vi "DLL Retcode to VI Errcode.vi"(8 "error in (no error)":errorcluster, 10 "Function Name":T1, 11 "DLL Retcode":i32 format="%x") -> (0 "error out":errorcluster, 2 "ErrorMessage":string, 3 "VI Errcode":i32 format="%x")   [LabVIEW 2020, in "Keyence CL-3000.lvlib"]
uses:
  Keyence CL-3000.lvlib
  enums/Function Name.ctl
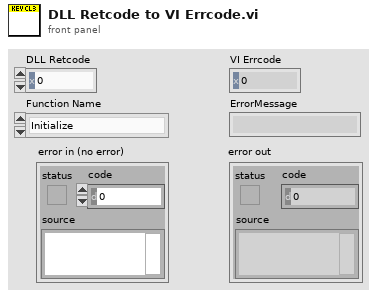
[diagram p1: front panel]
types:
  T1 = typedef "Keyence CL-3000.lvlib/Function Name.ctl" = enum16{"Initialize", "Close", "CL3IF_GetMeasurementData", "CL3IF_GetTrendIndex", "CL3IF_GetTrendData", "CL3IF_GetStorageIndex", "CL3IF_GetStorageData", "CL3IF_AutoZeroMulti", "CL3IF_AutoZeroGroup", "CL3IF_TimingMulti", "CL3IF_TimingGroup", "CL3IF_ResetMulti", "CL3IF_ResetGroup", "CL3IF_LightControl", "CL3IF_MeasurementControl", "CL3IF_SwitchProgram", "CL3IF_GetProgramNo", "CL3IF_StartStorage", "CL3IF_StopStorage", "CL3IF_ClearStorageData", "CL3IF_GetPulseCount", "CL3IF_ResetPulseCount", "CL3IF_GetLightWaveform"}
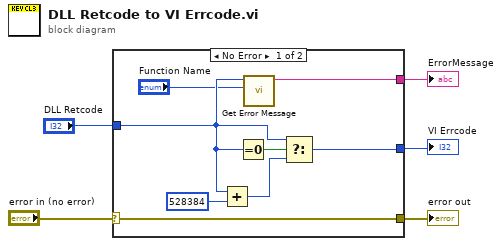
[diagram p0: block diagram]
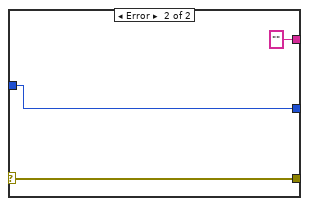
[diagram p2: hidden frame]
diagram:
  n1 = case shown="No Error" "error in (no error)" {
    selector: "error in (no error)" -> [w10 w15]
    tunnel: [w10 w15] -> w4
    tunnel: "DLL Retcode" -> [w8 w16]
    tunnel: [w9 w16] -> w2
    tunnel: [w6 "" ("ErrorMessage")] -> w1
    frame No Error {
      n2 = Add(x=w8, y=528384) -> (x+y=w11:i32)
      n3 = Equal To 0?(x=w8) -> (x = 0?=w13:bool)
      n4 = call "Get Error Message.vi"("Function Name"="Function Name", "DLL Retcode"=w8) -> ("ErrorMessage"=w6:string)  [unwired: 9 in]
      n5 = Select(t=w8, s=w13, f=w11) -> (s? t:f=w9:i32)
    }
    frame Error {
    }
  }
  "error out" <- w4
  "VI Errcode" <- w2
  "ErrorMessage" <- w1
